vi "QR-a.vi"(0 "Image In":T5, 1 "Image Dst":T5, 2 "ROI Descriptor (Pattern Matching 1)":T3={"Global Rectangle"=[20, 20, 890, 1177], "Contours"=[{"ID"=enum."External", "Type"=12, "Coordinates"=[20, 20, 890, 1177, 0]}]} {"Contours"."Type" items=["No Selection", "Point", "Line", "Rectangle", "Oval", "Polygon", "Freehand Region", "Annulus", "Unused2", "Unused3", "Broken Line", "Freehand Line", "Rotated Rectangle"]}, 3 "Algorithm (Pattern Matching 1)":i32(ring)=1 items=["All", "Low Discrepancy Sampling", "Grayscale Value Pyramid", "Gradients Pyramid"], 4 "Parameters (Pattern Matching 1)":T2={"Number of Matches Requested"=1, "Minimum Match Score"=400.0, "Angle Ranges"=[{"Start Angle"=-45.0, "End Angle"=45.0}]}, 5 "Advanced Options (Pattern Matching 1)":cluster{"Item":u16, "Value":dbl}[](array[cluster])=[{"Item"=0, "Value"=10.0}, {"Item"=2, "Value"=2.0}, {"Item"=5, "Value"=300.0}, {"Item"=6, "Value"=3.0}, {"Item"=7, "Value"=5.0}, {"Item"=8, "Value"=2.0}, {"Item"=1, "Value"=1.0}, {"Item"=3, "Value"=20.0}, {"Item"=4, "Value"=0.0}] {"Item" items=["LD Sampling - Minimum Constrast"=0, "LD Sampling - Enable Subpixel Accuracy"=1, "LD Sampling - Search Strategy"=2, "LD Sampling - Subpixel Iterations"=3, "LD Sampling - Subpixel Tolerance"=4, "LD Sampling - Initial Match List Length"=5, "LD Sampling - Match List Reduction Factor"=6, "LD Sampling - Initial Step Size"=7, "LD Sampling - Intermediate Angular Accuracy"=8, "-"=9, "Pyramid - Max Pyramid Level"=100, "Pyramid - Minimum Contrast"=102, "Pyramid - Enable Subpixel Accuracy"=103, "Pyramid - Subpixel Iterations"=104, "Pyramid - Subpixel Tolerance"=105, "Pyramid - Initial Match List Length"=106, "Pyramid - Match List Reduction Factor"=107, "Pyramid - Intermediate Angular Accuracy"=108, "Pyramid - Process Border Matches"=109, "Pyramid - Min Match Separation Distance"=111, "Pyramid - Min Match Separation Angle"=112, "Pyramid - Max Match Overlap"=113, "Pyramid - Max Cache in MB"=114, "Pyramid - Clear Cache"=115, "-"=116, "Enable Defect Map"=200]}, 6 "Template File Path (Pattern Matching 1)":path=path "D:/Inspect System/Source Code/SubVIs/字符检测VI/222.png", 7 "error in":errorcluster, 8 "QR Search Options (2D Barcode Reader 1)":T4={"Rotation Mode"=enum."Unlimited", "Skip Location?"=FALSE, "Edge Threshold"=11, "Demodulation Mode"=1, "Cell Sample Size"=3, "Cell Filter Mode"=2, "Skew Degrees Allowed"=5} {"Demodulation Mode" items=["Auto-detect"=-2, "Histogram"=0, "Local Contrast"=1, "Combination"=2, "All"=3]; "Cell Sample Size" items=["Auto-detect"=-2, "1x1"=1, "2x2"=2, "3x3"=3, "4x4"=4, "5x5"=5, "6x6"=6, "7x7"=7]; "Cell Filter Mode" items=["Auto-detect"=-2, "Average"=0, "Median"=1, "Central Average"=2, "High Average"=3, "Low Average"=4, "Very High Average"=5, "Very Low Average"=6, "All Filters"=8]}, 10 "ROI Descriptor (2D Barcode Reader 1)":T3={"Global Rectangle"=[579, 508, 906, 745], "Contours"=[{"ID"=enum."External", "Type"=3, "Coordinates"=[579, 508, 906, 745]}]} {"Contours"."Type" items=["No Selection", "Point", "Line", "Rectangle", "Oval", "Polygon", "Freehand Region", "Annulus", "Unused2", "Unused3", "Broken Line", "Freehand Line", "Rotated Rectangle"]}) -> (20 "Image Out":T5, 21 "Matches (Pattern Matching 1)":T14(array[cluster]) {"Bounding Box"."y" format="%.2f"; "Bounding Box"."x" format="%.2f"; "Position"."y" format="%.2f"; "Position"."x" format="%.2f"; "Score" format="%.2f"; "Scale" format="%.2f"; "Angle" format="%.2f"}, 22 "Calibrated Matches (Pattern Matching 1)":T14(array[cluster]) {"Bounding Box"."y" format="%.2f"; "Bounding Box"."x" format="%.2f"; "Position"."y" format="%.2f"; "Position"."x" format="%.2f"; "Score" format="%.2f"; "Scale" format="%.2f"; "Angle" format="%.2f"}, 23 "Number of Matches (Pattern Matching 1)":i32, 24 "Coordinate System Out (Set Coordinate System 1)":T13 {"Measurement System"."Axis Reference" items=["Direct", "Indirect"]; "Measurement System"."Angle (deg)" format="%.2f"; "Measurement System"."Origin"."Y" format="%.2f"; "Measurement System"."Origin"."X" format="%.2f"; "Reference System"."Axis Reference" items=["Direct", "Indirect"]; "Reference System"."Angle (deg)" format="%.2f"; "Reference System"."Origin"."Y" format="%.2f"; "Reference System"."Origin"."X" format="%.2f"}, 25 "Coordinate System Out":T1 {"Measurement System"."Axis Reference" items=["Direct", "Indirect"]; "Measurement System"."Angle (deg)" format="%.2f"; "Measurement System"."Origin"."Y" format="%.2f"; "Measurement System"."Origin"."X" format="%.2f"; "Reference System"."Axis Reference" items=["Direct", "Indirect"]; "Reference System"."Angle (deg)" format="%.2f"; "Reference System"."Origin"."Y" format="%.2f"; "Reference System"."Origin"."X" format="%.2f"}, 26 "QR Barcode Report (2D Barcode Reader 1)":T6={"Found?"=FALSE, "Data"="", "Bounding Box"=[], "Errors Corrected"=0, "Dimensions (Rows/Cols)"=0, "Version"=0, "QR Model"=3, "Stream Mode"=0, "Barcode Polarity"=-2, "Mirrored?"=FALSE, "Append Stream Position"=0, "Size of Append Stream"=0, "First EAN-128 ID"=0, "First Alternate Language ID"=0, "Append Stream ID"=0, "Minimum Edge Strength"=30, "Demodulation Mode"=-2, "Cell Sample Size"=-2, "Cell Filter Mode"=-2} {"Append Stream ID" format="%x"; "Cell Filter Mode" items=["Auto-detect"=-2, "Average"=0, "Median"=1, "Central Average"=2, "High Average"=3, "Low Average"=4, "Very High Average"=5, "Very Low Average"=6, "All Filters"=8]; "Cell Sample Size" items=["Auto-detect"=-2, "1x1"=1, "2x2"=2, "3x3"=3, "4x4"=4, "5x5"=5, "6x6"=6, "7x7"=7]; "Demodulation Mode" items=["Auto-detect"=-2, "Histogram"=0, "Local Contrast"=1, "Combination"=2, "All"=3]; "Barcode Polarity" items=["Auto-detect"=-2, "Black on White"=0, "White on Black"=1]; "Stream Mode" items=["Auto-detect", "Numeric", "AlphaNumeric", "Mixed", "Raw Bytes", "UCC/EAN-128 - In Tokens", "UCC/EAN-128 - In Data", "Extended Character Interpretation", "Kanji"]; "QR Model" items=["Auto Detect", "Micro", "Model 1", "Model 2"]; "Version" max=40 step=1}, 27 "error out":errorcluster)   [LabVIEW 2017]
doc: "Creates, edits, and runs vision algorithms using NI Vision Assistant.\n\nWhen you place this Express VI on the block diagram, NI Vision Assistant launches. Create an algorithm using the Vision Assistant processing functions. After you create an algorithm, you can select the controls and indicators that you want to be able to programmatically set in LabVIEW. Double-click the Vision Assistant Express VI to edit the algorithm."
uses:
  <vilib>/vision/Image Controls.llb/IMAQ Image.ctl
  <vilib>/vision/Instrument.llb/QR Code Report.ctl
  <vilib>/vision/Instrument.llb/QR Code Model Type.ctl
  <vilib>/vision/Instrument.llb/QR Code Stream Mode Type.ctl
  <vilib>/vision/Instrument.llb/Data Matrix Polarity.ctl
  <vilib>/vision/Instrument.llb/Demodulation Mode.ctl
  <vilib>/vision/Instrument.llb/Cell Sample Size.ctl
  <vilib>/vision/Instrument.llb/Cell Filter Mode.ctl
  <vilib>/vision/NI_Vision_Development_Module.lvlib
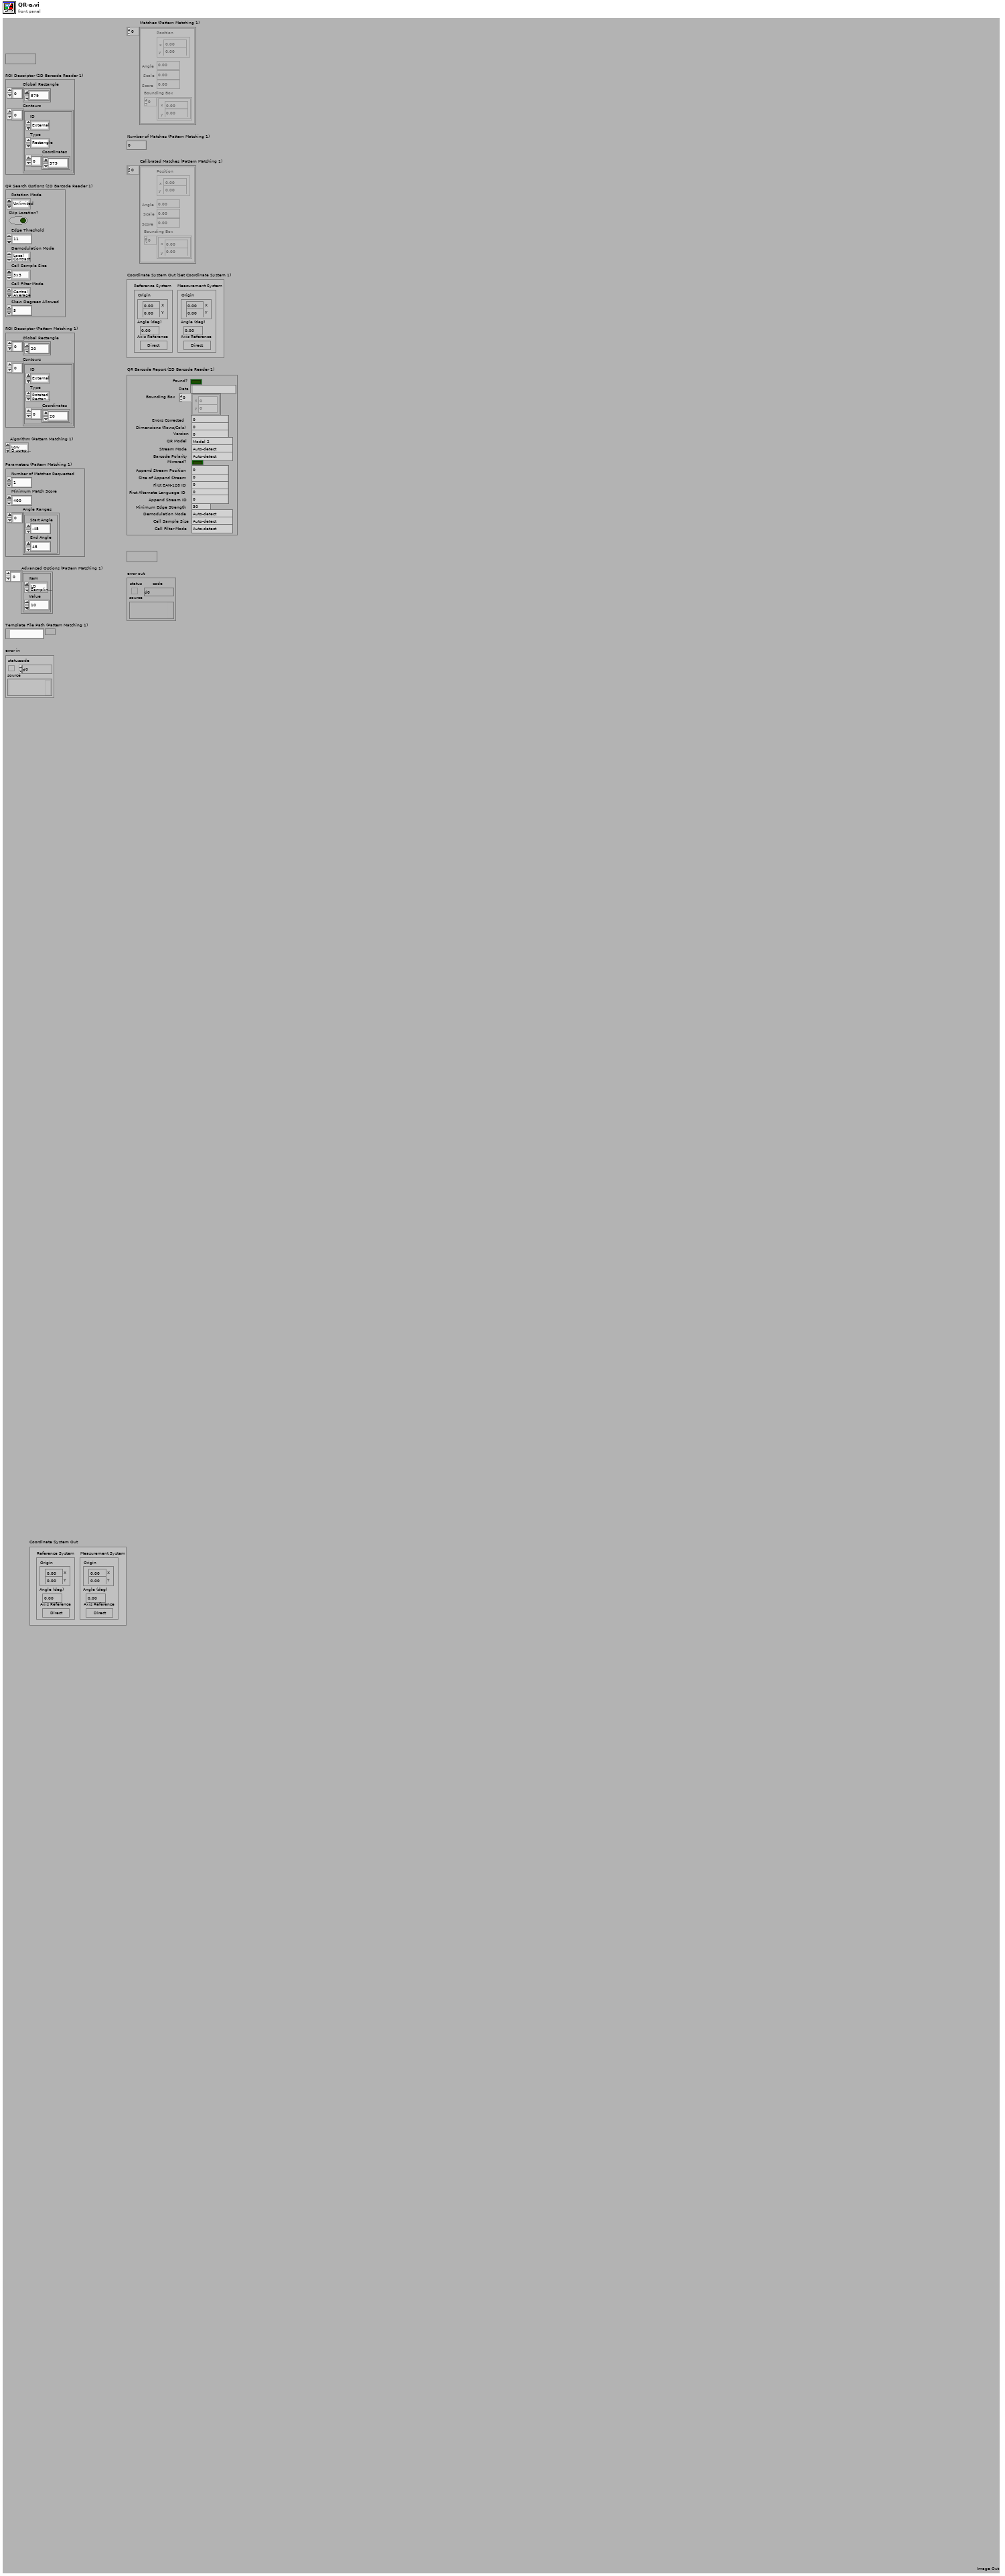
[diagram p1: front panel]
types:
  T1 = typedef "IMAQ Coordinate System" = cluster{"Reference System":cluster{"Origin":cluster{"X":sgl, "Y":sgl}, "Angle (deg)":sgl, "Axis Reference":u32}, "Measurement System":cluster{"Origin":cluster{"X":sgl, "Y":sgl}, "Angle (deg)":sgl, "Axis Reference":u32}}
  T2 = cluster{"Number of Matches Requested":i32, "Minimum Match Score":sgl, "Angle Ranges":cluster{"Start Angle":sgl, "End Angle":sgl}[]}
  T3 = cluster{"Global Rectangle":i32[], "Contours":cluster{"ID":enum32{"External", "Internal"}, "Type":u32, "Coordinates":i32[]}[]}
  T4 = cluster{"Rotation Mode":enum32{"Unlimited", "0 Degrees", "90 Degrees", "180 Degrees", "270 Degrees"}, "Skip Location?":bool, "Edge Threshold":u32, "Demodulation Mode":i32, "Cell Sample Size":i32, "Cell Filter Mode":i32, "Skew Degrees Allowed":u32}
  T5 = typedef "IMAQ Image.ctl" = refnum<image>
  T6 = typedef "QR Code Report.ctl" = cluster{"Found?":bool, "Data":string, "Bounding Box":cluster{"x":sgl, "y":sgl}[], "Errors Corrected":u32, "Dimensions (Rows/Cols)":u32, "Version":u32, "QR Model":T7, "Stream Mode":T8, "Barcode Polarity":T9, "Mirrored?":bool, "Append Stream Position":u32, "Size of Append Stream":u32, "First EAN-128 ID":i32, "First Alternate Language ID":i32, "Append Stream ID":u32, "Minimum Edge Strength":u32, "Demodulation Mode":T10, "Cell Sample Size":T11, "Cell Filter Mode":T12}
  T7 = typedef "QR Code Model Type.ctl" = i32
  T8 = typedef "QR Code Stream Mode Type.ctl" = i32
  T9 = typedef "Data Matrix Polarity.ctl" = i32
  T10 = typedef "Demodulation Mode.ctl" = i32
  T11 = typedef "Cell Sample Size.ctl" = i32
  T12 = typedef "Cell Filter Mode.ctl" = i32
  T13 = cluster{"Reference System":cluster{"Origin":cluster{"X":sgl, "Y":sgl}, "Angle (deg)":sgl, "Axis Reference":u32}, "Measurement System":cluster{"Origin":cluster{"X":sgl, "Y":sgl}, "Angle (deg)":sgl, "Axis Reference":u32}}
  T14 = cluster{"Position":cluster{"x":sgl, "y":sgl}, "Angle":sgl, "Scale":sgl, "Score":sgl, "Bounding Box":cluster{"x":sgl, "y":sgl}[]}[]
  T15 = cluster{"Origin":cluster{"X":sgl, "Y":sgl}, "Angle (deg)":sgl, "Axis Reference":u32}
  T16 = enum16{"Reset", "Update Coordinate System", "Get Coordinate System"}
  T17 = enum16{"Horizontal Motion", "Vertical Motion", "Horizontal and Vertical Motion", "Horizontal, Vertical and Angular Motion"}
  T18 = typedef "Image Type" = u32
  T19 = cluster{"Matrix Dimensions (cells)":i32, "Barcode Polarity":i32, "Mirror Mode":i32, "QR Model":i32}
  T20 = typedef "ROI Descriptor" = cluster{"Global Rectangle":i32[], "Contours":cluster{"ID":enum32{"External", "Internal"}, "Type":u32, "Coordinates":i32[]}[]}
  T21 = cluster{"Backup Image Name":string, "Coordinate System Out":T1}
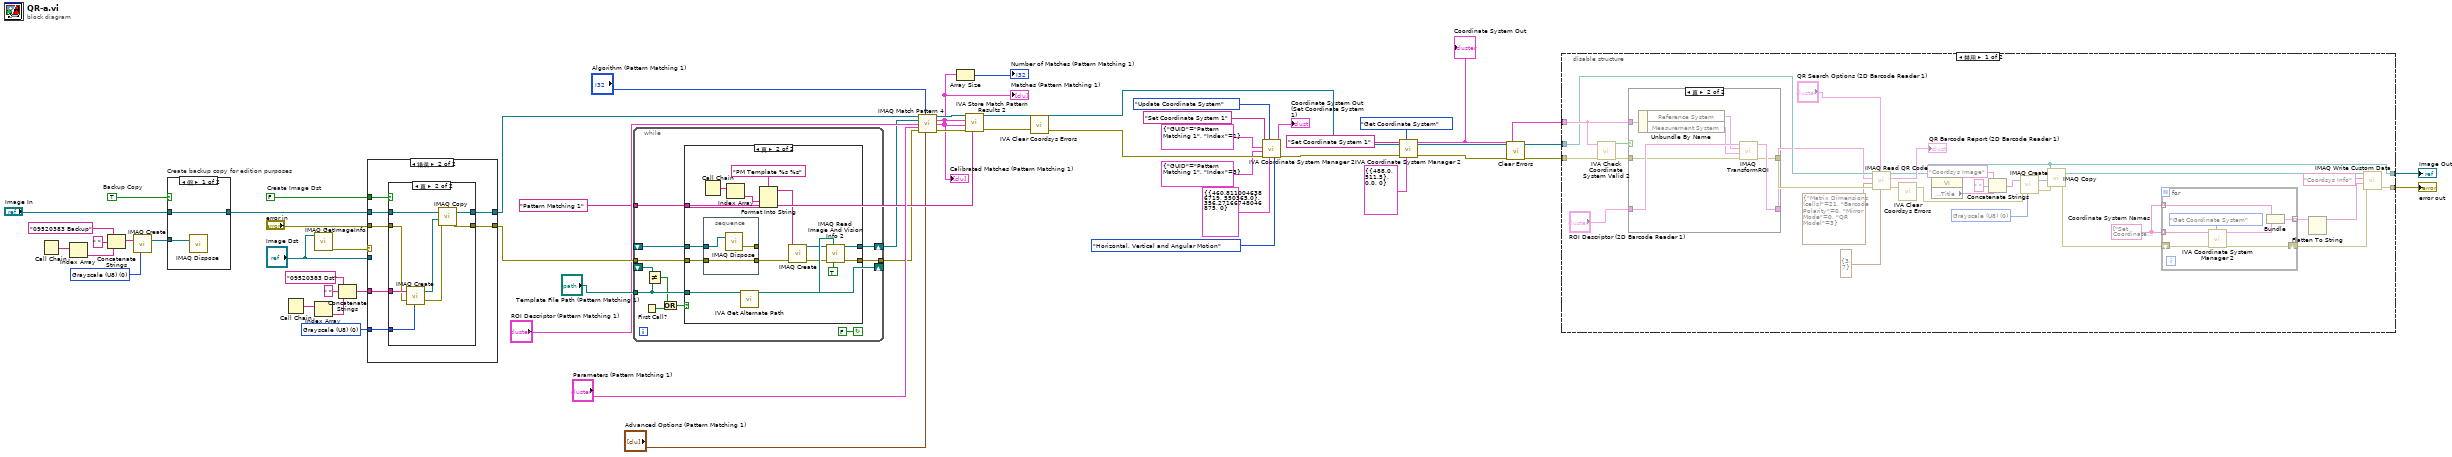
[diagram p0: block diagram]
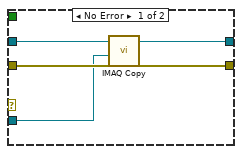
[diagram p5: hidden frame]
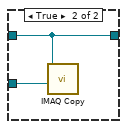
[diagram p7: hidden frame]
diagram:
  w25 = "Pattern Matching 1" ("Step Name")
  w34 = T18 0 items=["Grayscale (U8)", "Grayscale (I16)", "Grayscale (SGL)", "Complex (CSG)", "RGB (U32)", "HSL (U32)", "RGB (U64)", "Grayscale (U16)"] ("Image Dst Type")
  w35 = T18 0 items=["Grayscale (U8)", "Grayscale (I16)", "Grayscale (SGL)", "Complex (CSG)", "RGB (U32)", "HSL (U32)", "RGB (U64)", "Grayscale (U16)"] ("Image Type")
  w54 = TRUE  # Backup Copy
  w47 = FALSE  # Create Image Dst
  n1 = Call Chain() -> (call chain=w41:string[])
  n2 = Index Array(array=w41) -> (element=w40:string)  [unwired: 1 in]
  n3 = Concatenate Strings("09520383 Backup" ("Backup Image Name"), " ", w40) -> (w37:string)
  n4 = call "IMAQ Create"("Image Name"=w37, "Image Type"=w35) -> ("New Image"=w36:T5)  [unwired: 2 in, 2 out]
  n5 = case "Create backup copy for edition purposes" shown="假" w54 {
    tunnel: [w56 w58] -> w50
    tunnel: "Image In" -> [w56 w58]
    tunnel: w36 -> [w55 w57]
    frame False {
      n6 = call "IMAQ Dispose"("Image"=w55) -> ()  [unwired: 2 in, 4 out]
    }
    frame True {
      n7 = call "IMAQ Copy"("Image Dst"=w57, "Image Src"=w58) -> ()  [unwired: 1 in, 5 out]
    }
  }
  n8 = Call Chain() -> (call chain=w46:string[])
  n9 = call "IMAQ GetImageInfo"("Image"="Image Dst") -> ("error out"=w52:errorcluster)  [unwired: 1 in, 9 out]
  n10 = Index Array(array=w46) -> (element=w44:string)  [unwired: 1 in]
  n11 = Concatenate Strings("09520383 Dst" ("Image Dst Name"), " ", w44) -> (w42:string)
  n12 = case "条件结构" shown="错误" w52 {
    tunnel: [w63 w67] -> w32
    tunnel: [w62 w66] -> w48
    tunnel: w50 -> [w61 w68]
    tunnel: "error in" -> [w60 w64]
    tunnel: "Image Dst" -> [w59 _]
    tunnel: w42 -> [_ w70]
    tunnel: w34 -> [_ w69]
    tunnel: w47 -> [_ w65]
    frame No Error {
      n13 = call "IMAQ Copy"("error in (no error)"=w60, "Image Dst"=w59, "Image Src"=w61) -> ("error out"=w62:errorcluster, "Image Dst Out"=w63:T5)  [unwired: 3 out]
    }
    frame Error {
      n14 = case "条件结构" shown="真" w65 {
        tunnel: w70 -> [_ w80]
        tunnel: w69 -> [_ w79]
        tunnel: w68 -> [w72 w77]
        tunnel: [w72 w76] -> w67
        tunnel: [w71 w75] -> w66
        tunnel: w64 -> [w71 w73]
        frame False {
        }
        frame True {
          n15 = call "IMAQ Create"("Image Name"=w80, "Image Type"=w79, "error in (no error)"=w73) -> ("New Image"=w78:T5, "error out"=w74:errorcluster)  [unwired: 1 in, 1 out]
          n16 = call "IMAQ Copy"("error in (no error)"=w74, "Image Dst"=w78, "Image Src"=w77) -> ("error out"=w75:errorcluster, "Image Dst Out"=w76:T5)  [unwired: 3 out]
        }
      }
    }
  }
  n17 = while {
    shift-right: [w91] -> w22
    shift-left: _ -> [w90]
    tunnel: [w88] -> w21
    tunnel: w48 -> [w87]
    tunnel: "Template File Path (Pattern Matching 1)" -> [w84]
    tunnel: w25 -> [w86]
    shift-right: [w84] -> _
    shift-left: _ -> [w85]
    stop <- FALSE continue-if-true
    n18 = First Call?() -> (First Call?: T/F=w83:bool)
    n19 = Not Equal?(x=w85, y=w84) -> (x != y?=w82:bool)
    n20 = Or(x=w82, y=w83) -> (x .or. y?=w81:bool)
    n21 = case "条件结构" shown="真" w81 {
      tunnel: [w93 w98] -> w91
      tunnel: w90 -> [w93 w102]
      tunnel: [w92 w99] -> w88
      tunnel: w87 -> [w92 w101]
      tunnel: w84 -> [_ w103]
      tunnel: w86 -> [_ w104]
      frame False {
      }
      frame True {
        n22 = stacked-sequence "层叠式顺序结构" {
          tunnel: w102 -> [w111]
          tunnel: w101 -> [w110]
          tunnel: [w110] -> w95
          tunnel: [w109] -> _
          frame #0 {
            n23 = call "IMAQ Dispose"("Image"=w111) -> ("error out"=w109:errorcluster)  [unwired: 2 in, 3 out]
          }
        }
        n24 = Call Chain() -> (call chain=w106:string[])
        n25 = Index Array(array=w106) -> (element=w105:string)  [unwired: 1 in]
        n26 = call <vilib>:"IVA Get Alternate Path.vi"("Path In"=w103) -> ("Path Out"=w100:path)  [unwired: 10 out]
        n27 = Format Into String(format string="PM Template %s %s" ("Image Name"), w105, w104) -> (resulting string=w108:string)  [unwired: 2 in, 1 out]
        n28 = call "IMAQ Create"("Image Name"=w108, "error in (no error)"=w95) -> ("New Image"=w97:T5, "error out"=w96:errorcluster)  [unwired: 2 in, 1 out]
        n29 = call "IMAQ Read Image And Vision Info 2"("Use File Path Image Type"=TRUE, "File Path"=w100, "error in (no error)"=w96, "Image"=w97) -> ("error out"=w99:errorcluster, "Image Out"=w98:T5)  [unwired: 5 in, 1 out]
      }
    }
  }
  n30 = call "IMAQ Match Pattern 4"("Image"=w32, "Algorithm"="Algorithm (Pattern Matching 1)", "Template Image"=w22, "ROI Descriptor"="ROI Descriptor (Pattern Matching 1)", "Parameters"="Parameters (Pattern Matching 1)", "error in (no error)"=w21, "Advanced Options"="Advanced Options (Pattern Matching 1)") -> ("Image (duplicate)"=w30:T5, "Matches (pixel)"=w24:T14, "Matches (real-world)"=w23:T14, "error out"=w31:errorcluster)  [unwired: 4 in, 1 out]
  "Matches (Pattern Matching 1)" <- w24
  "Calibrated Matches (Pattern Matching 1)" <- w23
  n31 = Array Size(array=w24) -> (size(s)=→"Number of Matches (Pattern Matching 1)":i32)
  n32 = call <vilib>:"IVA Store Match Pattern Results 2.vi"("Step Name"=w25, "error in (no error)"=w31, "Matches (real-world)"=w23, "Matches (pixel)"=w24, "Image in"=w30) -> ("error out"=w20:errorcluster, "Image dup"=w4:T5)  [unwired: 1 in, 4 out]
  n33 = call <vilib>:"IVA Clear Coordsys Errors.vi"("error in (no error)"=w20) -> ("error out"=w19:errorcluster)  [unwired: 10 in]
  n34 = call <vilib>:"IVA Coordinate System Manager 2.vi"("Mode"=T17."Horizontal, Vertical and Angular Motion", "Reference System"=T15 {"Origin"={"X"=460.811, "Y"=550365.0}, "Angle (deg)"=356.27167, "Axis Reference"=0}, "Function"=T16."Update Coordinate System", "error in (no error)"=w19, "Angle ID"=cluster{"GUID":string, "Index":i32} {"GUID"="Pattern Matching 1", "Index"=3}, "Origin ID"=cluster{"GUID":string, "Index":i32} {"GUID"="Pattern Matching 1", "Index"=1}, "Coordinate System Name"="Set Coordinate System 1") -> ("error out"=w11:errorcluster, "Coordinate System Out"=→"Coordinate System Out (Set Coordinate System 1)":T1)  [unwired: 3 out]
  n35 = call <vilib>:"IVA Coordinate System Manager 2.vi"("Reference System"=T15 {"Origin"={"X"=488.0, "Y"=511.5}, "Angle (deg)"=0.0, "Axis Reference"=0}, "Function"=T16."Get Coordinate System", "error in (no error)"=w11, "Coordinate System Name"="Set Coordinate System 1") -> ("error out"=w7:errorcluster, "Coordinate System Out"=w5:T1)  [unwired: 3 in, 3 out]
  "Coordinate System Out" <- w5
  n36 = call <vilib>:"Clear Errors.vi"("error in (no error)"=w7) -> ("error out"=w1:errorcluster)  [unwired: 5 in, 1 out]
  n37 = disable-structure shown="禁用" {
    disable-tunnel: w5 -> [w139 _]
    disable-tunnel: w4 -> [w136 w159]
    disable-tunnel: [w119 w158] -> w3
    disable-tunnel: [w113 w159] -> w2
    disable-tunnel: w1 -> [w112 w158]
    frame Disabled {
      w116 = T18 0 items=["Grayscale (U8)", "Grayscale (I16)", "Grayscale (SGL)", "Complex (CSG)", "RGB (U32)", "HSL (U32)", "RGB (U64)", "Grayscale (U16)"] ("Image Type")
      w123 = string[] ["Set Coordinate System 1"]  # Coordinate System Names
      n38 = call <vilib>:"IVA Check Coordinate System Valid 2.vi"("error in (no error)"=w112, "Coordinate System"=w139) -> ("error out"=w137:errorcluster, "Valid?"=w138:bool)  [unwired: 8 out]
      n39 = case "条件结构" shown="真" w138 {
        tunnel: "ROI Descriptor (2D Barcode Reader 1)" -> [w150 w157]
        tunnel: [w150 w154] -> w131
        tunnel: [w149 w153] -> w140
        tunnel: w139 -> [_ w152]
        tunnel: w137 -> [w149 w151]
        frame False {
        }
        frame True {
          n40 = Unbundle By Name(w152) -> ("Reference System"=w156:T15, "Measurement System"=w155:T15)
          n41 = call "IMAQ TransformROI"("error in (no error)"=w151, "New Reference"=w155, "Base Reference"=w156, "ROI Descriptor"=w157) -> ("error out"=w153:errorcluster, "ROI Descriptor out"=w154:T20)  [unwired: 6 out]
        }
      }
      n42 = call "IMAQ Read QR Code"("QR Code Cell Size (pixels)"=cluster{"Minimum Size":u32, "Maximum Size":u32} {"Minimum Size"=3, "Maximum Size"=7}, "QR Search Options"="QR Search Options (2D Barcode Reader 1)", "error in (no error)"=w140, "QR Description Options"=T19 {"Matrix Dimensions (cells)"=21, "Barcode Polarity"=0, "Mirror Mode"=0, "QR Model"=3}, "ROI Descriptor"=w131, "Image"=w136) -> ("error out"=w130:errorcluster, "QR Code Report"=→"QR Barcode Report (2D Barcode Reader 1)":T6, "Image (duplicate)"=w113:T5)  [unwired: 1 in, 2 out]
      n43 = call <vilib>:"IVA Clear Coordsys Errors.vi"("error in (no error)"=w130) -> ("error out"=w129:errorcluster)  [unwired: 10 in]
      n44 = property class="VI"() -> ("Front Panel Window:Title"=w117:string)  [unwired: 2 in, 2 out]
      n45 = Concatenate Strings("Coordsys Image" ("Processed Image Name"), " ", w117) -> (w126:string)
      n46 = call "IMAQ Create"("Image Name"=w126, "Image Type"=w116, "error in (no error)"=w129) -> ("New Image"=w124:T5, "error out"=w125:errorcluster)  [unwired: 1 in, 1 out]
      n47 = call "IMAQ Copy"("error in (no error)"=w125, "Image Dst"=w124, "Image Src"=w113) -> ("error out"=w115:errorcluster, "Image Dst Out"=w122:T5)  [unwired: 3 out]
      n48 = for "For循环" {
        tunnel: w123 -> [w147] mode=indexing
        tunnel: w123 -> [w145] mode=indexing
        tunnel: [w144] -> w121 mode=indexing
        shift-right: [w142] -> w114
        shift-left: w115 -> [w143]
        n49 = call <vilib>:"IVA Coordinate System Manager 2.vi"("Function"=T16."Get Coordinate System", "error in (no error)"=w143, "Coordinate System Name"=w147) -> ("error out"=w142:errorcluster, "Coordinate System Out"=w146:T1)  [unwired: 4 in, 3 out]
        n50 = Bundle("Backup Image Name"=w145, "Coordinate System Out"=w146) -> (w144:T21)  [unwired: 1 out]
      }
      n51 = Flatten To String(anything=w121) -> (data string=w120:string)  [unwired: 1 in, 4 out]
      n52 = call "IMAQ Write Custom Data"("error in (no error)"=w114, "Custom Data In"=w120, "Key"="Coordsys Info", "Image"=w122) -> ("error out"=w119:errorcluster)  [unwired: 7 out]
    }
    frame Enabled {
    }
  }
  "error out" <- w3
  "Image Out" <- w2
